vi "PosEchoTableToSimpeTable.vi"(5 "Convert To Simple Table":bool, 7 "UpdateToRealSubcode(T=Real)":bool, 8 "error constant IN":errorcluster, 11 "RawPosEchoTable":string[][](array[string])) -> (0 "error out":errorcluster, 2 "TagList":string[](array[string]), 3 "SimplePosTable":string[][](array[string]))   [LabVIEW 2011]
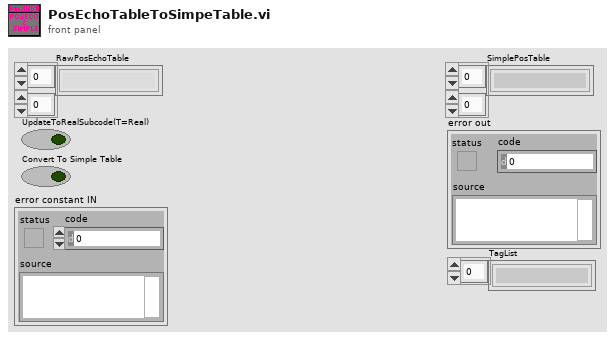
[diagram p1: front panel]
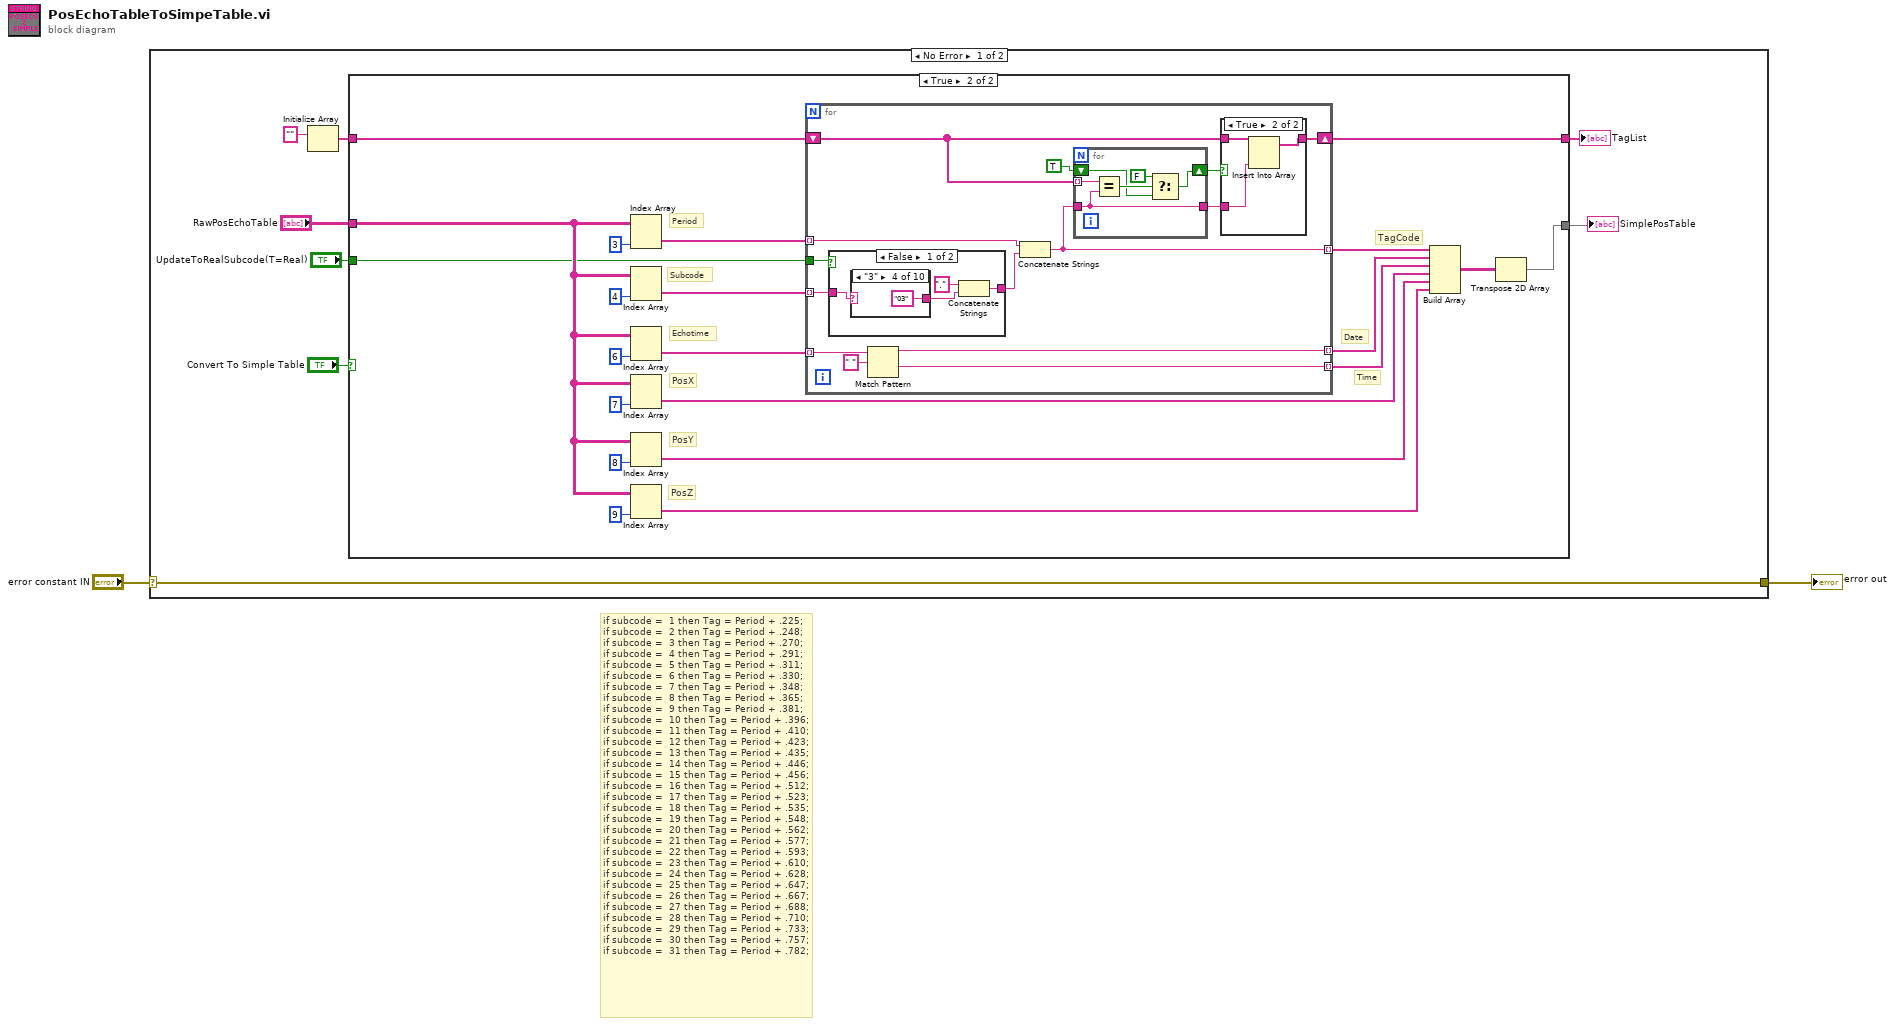
[diagram p0: block diagram]
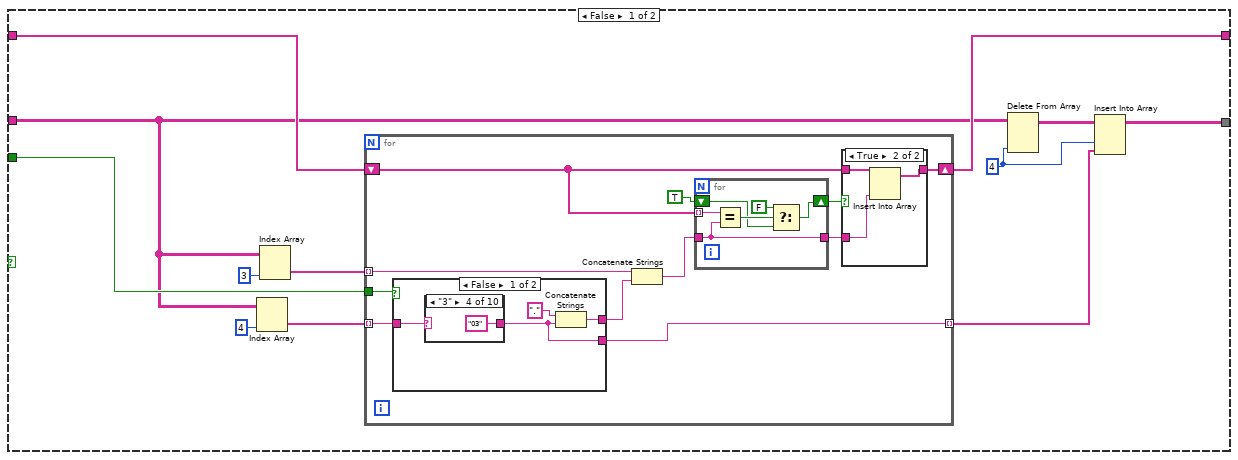
[diagram p2: hidden frame]
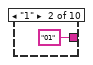
[diagram p5: hidden frame]
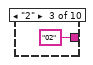
[diagram p6: hidden frame]
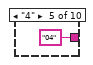
[diagram p7: hidden frame]
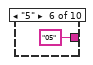
[diagram p8: hidden frame]
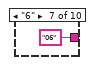
[diagram p9: hidden frame]
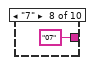
[diagram p10: hidden frame]
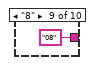
[diagram p11: hidden frame]
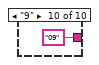
[diagram p12: hidden frame]
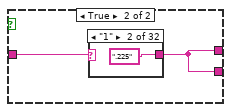
[diagram p13: hidden frame]
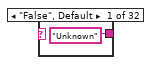
[diagram p14: hidden frame]
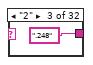
[diagram p15: hidden frame]
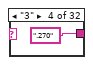
[diagram p16: hidden frame]
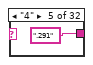
[diagram p17: hidden frame]
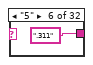
[diagram p18: hidden frame]
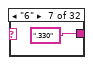
[diagram p19: hidden frame]
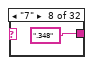
[diagram p20: hidden frame]
diagram:
  # "if subcode = \t1\tthen Tag =\tPeriod + .225;\nif subcode = \t2\tthen Tag =\tPeriod + .248;\nif subcode = \t3\tthen Tag =\tPeriod + .270;\nif subcode = \t4\tthen Tag =\tPeriod + .291;\nif subcode = \t5\tthen Tag =\tPeriod + .311;\nif subcode = \t6\tthen Tag =\tPeriod + .330;\nif subcode = \t7\tthen Tag =\tPeriod + .348;\nif subcode = \t8\tthen Tag =\tPeriod + .365;\nif subcode = \t9\tthen Tag =\tPeriod + .381;\nif subcode = \t10\tthen Tag =\tPeriod + .396;\nif subcode = \t11\tthen Tag =\tPeriod + .410;\nif subcode = \t12\tthen Tag =\tPeriod + .423;\nif subcode = \t13\tthen Tag =\tPeriod + .435;\nif subcode = \t14\tthen Tag =\tPeriod + .446;\nif subcode = \t15\tthen Tag =\tPeriod + .456;\nif subcode = \t16\tthen Tag =\tPeriod + .512;\nif subcode = \t17\tthen Tag =\tPeriod + .523;\nif subcode = \t18\tthen Tag =\tPeriod + .535;\nif subcode = \t19\tthen Tag =\tPeriod + .548;\nif subcode = \t20\tthen Tag =\tPeriod + .562;\nif subcode = \t21\tthen Tag =\tPeriod + .577;\nif subcode = \t22\tthen Tag =\tPeriod + .593;\nif subcode = \t23\tthen Tag =\tPeriod + .610;\nif subcode = \t24\tthen Tag =\tPeriod + .628;\nif subcode = \t25\tthen Tag =\tPeriod + .647;\nif subcode = \t26\tthen Tag =\tPeriod + .667;\nif subcode = \t27\tthen Tag =\tPeriod + .688;\nif subcode = \t28\tthen Tag =\tPeriod + .710;\nif subcode = \t29\tthen Tag =\tPeriod + .733;\nif subcode = \t30\tthen Tag =\tPeriod + .757;\nif subcode = \t31\tthen Tag =\tPeriod + .782;"
  n1 = case shown="No Error" "error constant IN" {
    selector: "error constant IN" -> [w8 w185]
    tunnel: [w8 w185] -> w1
    frame No Error {
      n2 = Initialize Array("") -> (w6:string[])  [unwired: 1 in]
      n3 = case shown="True" "Convert To Simple Table" {
        tunnel: "RawPosEchoTable" -> [w15 w97]
        tunnel: [w13 w92] -> w3
        tunnel: w6 -> [w18 w96]
        tunnel: [w17 w95] -> w5
        tunnel: "UpdateToRealSubcode(T=Real)" -> [w16 w94]
        frame False {
          w11 = 4 ("disabled index (col)")
          n4 = Index Array(array=w15, index (col)=4 ("disabled index (col)")) -> (element=w19:string[])  [unwired: 1 in]
          n5 = Index Array(array=w15, index (col)=3 ("disabled index (col)")) -> (element=w21:string[])  [unwired: 1 in]
          n6 = for {
            tunnel: w21 -> [w26] mode=indexing
            tunnel: w19 -> [w33] mode=indexing
            tunnel: w16 -> [w32]
            shift-right: [w28] -> w17
            shift-left: w18 -> [w29]
            tunnel: [w24] -> w12 mode=indexing
            n7 = case shown="False" w32 {
              tunnel: w33 -> [w45 w59]
              tunnel: [w47 w58] -> w23
              tunnel: [w44 w58] -> w24
              frame False {
                n8 = case shown="\"3\"" w45 {
                  selector: w45 -> [w48 _ _ _ _ _ _ _ _ _]
                  tunnel: [w48 "01" "02" "03" "04" "05" "06" "07" "08" "09"] -> w44
                  frame "False", Default {
                  }
                  frame "1" {
                  }
                  frame "2" {
                  }
                  frame "3" {
                  }
                  frame "4" {
                  }
                  frame "5" {
                  }
                  frame "6" {
                  }
                  frame "7" {
                  }
                  frame "8" {
                  }
                  frame "9" {
                  }
                }
                n9 = Concatenate Strings("." ("string"), w44) -> (w47:string)
              }
              frame True {
                n10 = case shown="\"1\"" w59 {
                  tunnel: ["Unknown" ".225" ".248" ".270" ".291" ".311" ".330" ".348" ".365" ".381" ".396" ".410" ".423" ".435" ".446" ".456" ".512" ".523" ".535" ".548" ".562" ".577" ".593" ".610" ".628" ".647" ".667" ".688" ".710" ".733" ".757" ".782"] -> w58
                  frame "False", Default {
                  }
                  frame "1" {
                  }
                  frame "2" {
                  }
                  frame "3" {
                  }
                  frame "4" {
                  }
                  frame "5" {
                  }
                  frame "6" {
                  }
                  frame "7" {
                  }
                  frame "8" {
                  }
                  frame "9" {
                  }
                  frame "10" {
                  }
                  frame "11" {
                  }
                  frame "12" {
                  }
                  frame "13" {
                  }
                  frame "14" {
                  }
                  frame "15" {
                  }
                  frame "16" {
                  }
                  frame "17" {
                  }
                  frame "18" {
                  }
                  frame "19" {
                  }
                  frame "20" {
                  }
                  frame "21" {
                  }
                  frame "22" {
                  }
                  frame "23" {
                  }
                  frame "24" {
                  }
                  frame "25" {
                  }
                  frame "26" {
                  }
                  frame "27" {
                  }
                  frame "28" {
                  }
                  frame "29" {
                  }
                  frame "30" {
                  }
                  frame "31" {
                  }
                }
              }
            }
            n11 = Concatenate Strings(w26, w23) -> (w25:string)
            n12 = for {
              tunnel: w29 -> [w43] mode=indexing
              tunnel: w25 -> [w38]
              shift-right: [w42] -> w30
              shift-left: TRUE -> [w40]
              tunnel: [w38] -> w27
              n13 = Equal?(x=w43, y=w38) -> (x = y?=w41:bool)
              n14 = Select(t=FALSE, s=w41, f=w40) -> (s? t:f=w42:bool)
            }
            n15 = case shown="True" w30 {
              tunnel: w29 -> [w34 w37]
              tunnel: [w34 w36] -> w28
              tunnel: w27 -> [_ w35]
              frame False {
              }
              frame True {
                n16 = Insert Into Array(array=w37, new element=w35) -> (w36:string[])  [unwired: 1 in]
              }
            }
          }
          n17 = Delete From Array(array=w15, index (col)=w11) -> (array with subset deleted=w14:string[][])  [unwired: 2 in, 1 out]
          n18 = Insert Into Array(array=w14, index (col)=w11, new element=w12) -> (w13:string[][])  [unwired: 1 in]
        }
        frame True {
          # "Time"
          # "Date"
          # "TagCode"
          # "PosZ"
          # "PosY"
          # "PosX"
          # "Echotime"
          # "Subcode"
          # "Period"
          n19 = Index Array(array=w97, index (col)=3 ("disabled index (col)")) -> (element=w103:string[])  [unwired: 1 in]
          n20 = Index Array(array=w97, index (col)=4 ("disabled index (col)")) -> (element=w102:string[])  [unwired: 1 in]
          n21 = Index Array(array=w97, index (col)=6 ("disabled index (col)")) -> (element=w100:string[])  [unwired: 1 in]
          n22 = Index Array(array=w97, index (col)=7 ("disabled index (col)")) -> (element=w106:string[])  [unwired: 1 in]
          n23 = Index Array(array=w97, index (col)=8 ("disabled index (col)")) -> (element=w105:string[])  [unwired: 1 in]
          n24 = Index Array(array=w97, index (col)=9 ("disabled index (col)")) -> (element=w104:string[])  [unwired: 1 in]
          n25 = for {
            tunnel: w103 -> [w124] mode=indexing
            tunnel: w102 -> [w126] mode=indexing
            tunnel: w94 -> [w125]
            tunnel: [w118] -> w101 mode=indexing
            tunnel: w100 -> [w122] mode=indexing
            tunnel: [w120] -> w99 mode=indexing
            tunnel: [w119] -> w98 mode=indexing
            shift-right: [w114] -> w95
            shift-left: w96 -> [w115]
            n26 = case shown="False" w125 {
              tunnel: w126 -> [w138 w152]
              tunnel: [w140 w151] -> w123
              frame False {
                n27 = case shown="\"3\"" w138 {
                  selector: w138 -> [w141 _ _ _ _ _ _ _ _ _]
                  tunnel: [w141 "01" "02" "03" "04" "05" "06" "07" "08" "09"] -> w137
                  frame "False", Default {
                  }
                  frame "1" {
                  }
                  frame "2" {
                  }
                  frame "3" {
                  }
                  frame "4" {
                  }
                  frame "5" {
                  }
                  frame "6" {
                  }
                  frame "7" {
                  }
                  frame "8" {
                  }
                  frame "9" {
                  }
                }
                n28 = Concatenate Strings("." ("string"), w137) -> (w140:string)
              }
              frame True {
                n29 = case shown="\"15\"" w152 {
                  tunnel: ["Unknown" ".225" ".248" ".270" ".291" ".311" ".330" ".348" ".365" ".381" ".396" ".410" ".423" ".435" ".446" ".456" ".512" ".523" ".535" ".548" ".562" ".577" ".593" ".610" ".628" ".647" ".667" ".688" ".710" ".733" ".757" ".782"] -> w151
                  frame "False", Default {
                  }
                  frame "1" {
                  }
                  frame "2" {
                  }
                  frame "3" {
                  }
                  frame "4" {
                  }
                  frame "5" {
                  }
                  frame "6" {
                  }
                  frame "7" {
                  }
                  frame "8" {
                  }
                  frame "9" {
                  }
                  frame "10" {
                  }
                  frame "11" {
                  }
                  frame "12" {
                  }
                  frame "13" {
                  }
                  frame "14" {
                  }
                  frame "15" {
                  }
                  frame "16" {
                  }
                  frame "17" {
                  }
                  frame "18" {
                  }
                  frame "19" {
                  }
                  frame "20" {
                  }
                  frame "21" {
                  }
                  frame "22" {
                  }
                  frame "23" {
                  }
                  frame "24" {
                  }
                  frame "25" {
                  }
                  frame "26" {
                  }
                  frame "27" {
                  }
                  frame "28" {
                  }
                  frame "29" {
                  }
                  frame "30" {
                  }
                  frame "31" {
                  }
                }
              }
            }
            n30 = Match Pattern(string=w122, regular expression=" ") -> (before substring=w120:string, after substring=w119:string)  [unwired: 1 in, 2 out]
            n31 = Concatenate Strings(w124, w123) -> (w118:string)
            n32 = for {
              tunnel: w115 -> [w136] mode=indexing
              tunnel: w118 -> [w131]
              shift-right: [w135] -> w116
              shift-left: TRUE -> [w133]
              tunnel: [w131] -> w113
              n33 = Equal?(x=w136, y=w131) -> (x = y?=w134:bool)
              n34 = Select(t=FALSE, s=w134, f=w133) -> (s? t:f=w135:bool)
            }
            n35 = case shown="True" w116 {
              tunnel: w115 -> [w127 w130]
              tunnel: [w127 w129] -> w114
              tunnel: w113 -> [_ w128]
              frame False {
              }
              frame True {
                n36 = Insert Into Array(array=w130, new element=w128) -> (w129:string[])  [unwired: 1 in]
              }
            }
          }
          n37 = Build Array(w101, w99, w98, w106, w105, w104) -> (w93:string[][])
          n38 = Transpose 2D Array(2D array=w93) -> (transposed array=w92:string[][])
        }
      }
      "SimplePosTable" <- w3
      "TagList" <- w5
    }
    frame Error {
    }
  }
  "error out" <- w1
